vi "4AHMBA.vi"() -> ()   [LabVIEW 2012]
uses:
  <vilib>/express/express shared/transition.llb/Dynamic To Waveform Array.vi
  <vilib>/express/express shared/transition.llb/Waveform Array To Dynamic.vi
  <vilib>/express/express arith-compare/Formula/Block/exnFormulaBlock how many pts in the wave.vi
  <vilib>/express/express shared/ex_Modify Signal Name.vi
  <vilib>/express/express arith-compare/Formula/XNode/ExpressFormulaBlockNode.xnode
panel:
  out "cw - Wert":dbl
  out "cw - Wert":dynamicdata(graph)
  out "v in [m/s]":dbl
  out "F in [N]":dbl
  out "F in [N]":dynamicdata(graph)
  out "v in [m/s]":dynamicdata(graph)
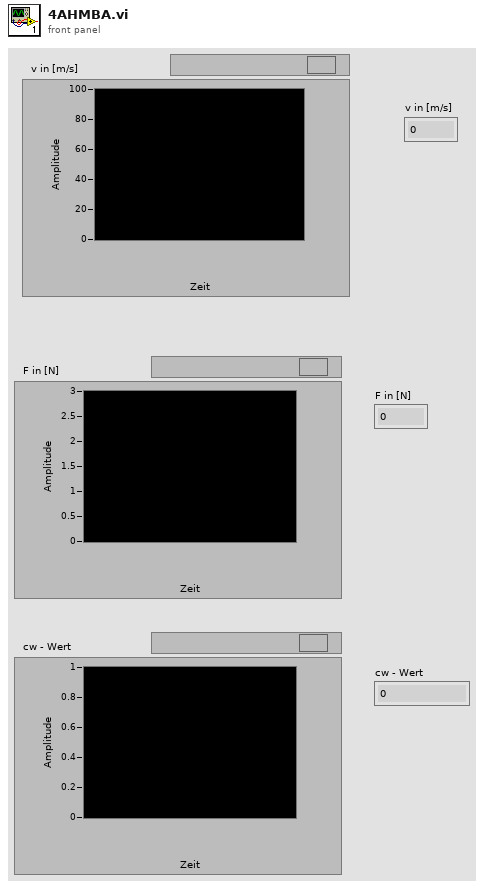
[diagram p1: front panel]
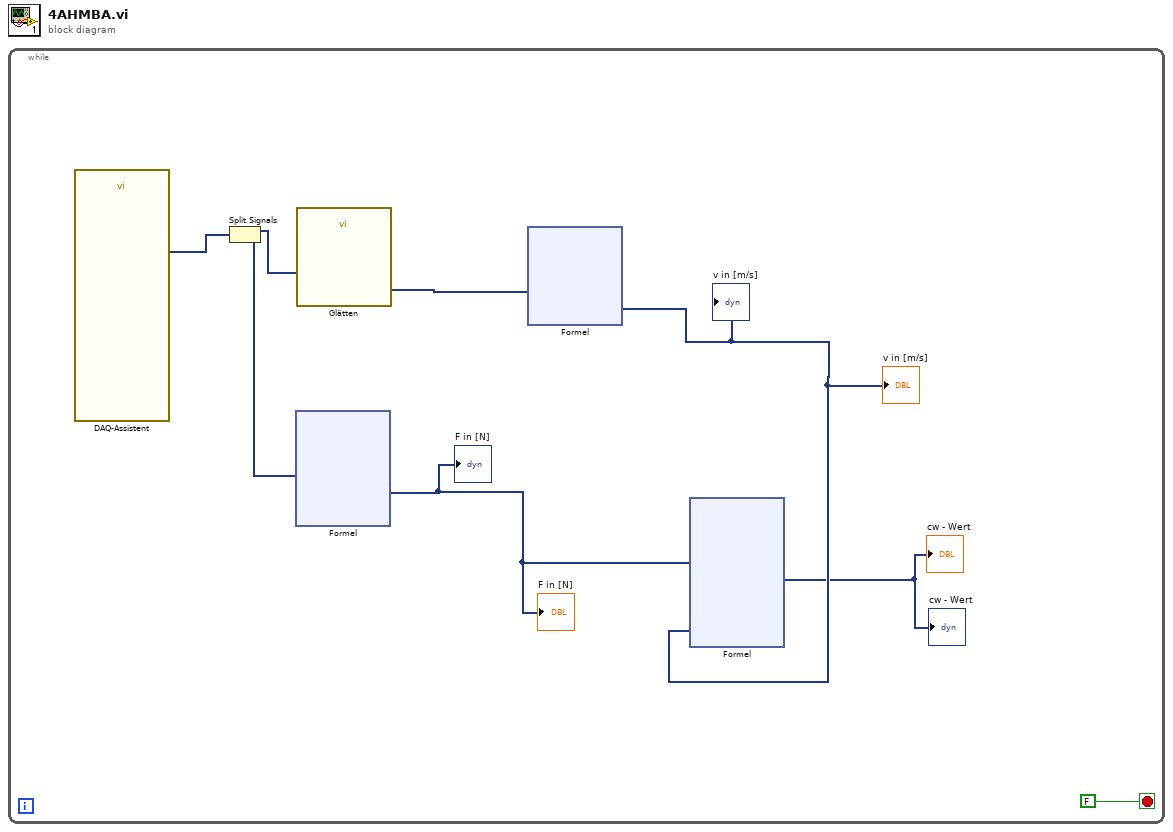
[diagram p0: block diagram]
diagram:
  n1 = while {
    stop <- FALSE stop-if-true
    n2 = call "DAQ-Assistent"() -> ("data"=w7:dynamicdata)  [unwired: 16 in, 3 out]
    n3 = Split Signals(w7) -> (w5:dynamicdata, w6:dynamicdata)  [unwired: 2 in]
    n4 = xnode "Formel"("X1"=w6) -> ("Ergebnis"=w3:dynamicdata)  [unwired: 1 in, 1 out]
    "F in [N]" <- w3
    "F in [N]" <- w3
    n5 = call "Glätten"("Signal"=w5) -> ("Filtered Signal"=w4:dynamicdata)  [unwired: 9 in, 1 out]
    n6 = xnode "Formel"("X1"=w4) -> ("Ergebnis"=w2:dynamicdata)  [unwired: 1 in, 1 out]
    "v in [m/s]" <- w2
    "v in [m/s]" <- w2
    n7 = xnode "Formel"("F"=w3, "v"=w2) -> ("Ergebnis"=→"cw - Wert" →"cw - Wert":dynamicdata)  [unwired: 1 in, 1 out]
  }
